vi "From Variant.vi"(8 "error in (no error)":errorcluster, 10 "Variant":variant, 11 "Abs_Time in":refnum<class "Abs_Time 1D.lvclass">) -> (0 "error out":errorcluster, 3 "Abs_Time out":refnum<class "Abs_Time 1D.lvclass">)   [LabVIEW 2021, in "Abs_Time 1D.lvclass"]
uses:
  Abs_Time 1D.lvclass
  Support/Type.ctl
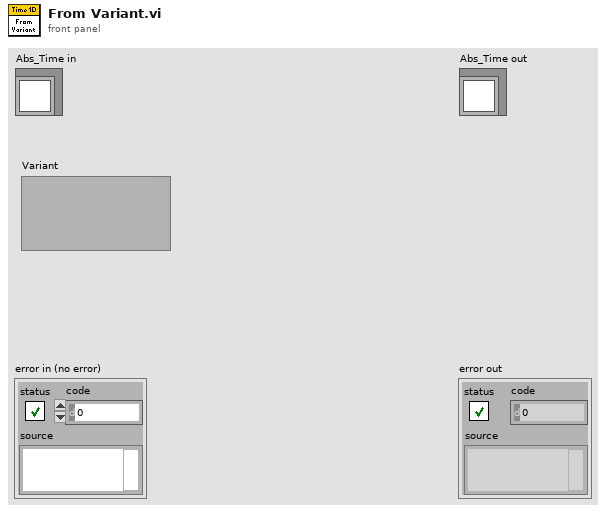
[diagram p1: front panel]
types:
  T1 = typedef "Abs_Time 1D.lvclass/Type.ctl" = timestamp[]
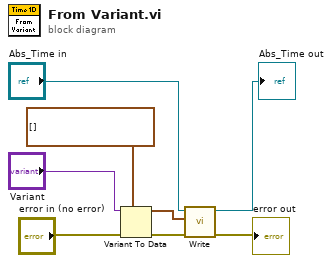
[diagram p0: block diagram]
diagram:
  n1 = Variant To Data(error in="error in (no error)", type=T1 [], Variant="Variant") -> (data=w5:T1, error out=w6:errorcluster)
  n2 = call-dynamic "Write.vi"("error in (no error)"=w6, "Value"=w5, "Double Float.lvclass_340760 in"="Abs_Time in") -> ("error out"=→"error out":errorcluster, "Double Float.lvclass_340760 out"=→"Abs_Time out":refnum<class "Abs_Time 1D.lvclass">)  [unwired: 7 in]
